vi "Create Object.vi"(11 "Ex Event Actor in":refnum<class "Ex Event Actor.lvclass">) -> (3 "Ex Event Actor out":refnum<class "Ex Event Actor.lvclass">)   [LabVIEW 2021, in "Ex Event Actor.lvclass"]
uses:
  Ex Event Actor.lvclass
  Ex Event Actor.lvclass/Ex Event Actor.ctl
  jettl/jettl.lvlib
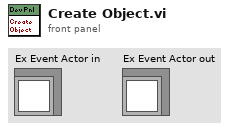
[diagram p1: front panel]
types:
  T1 = cluster{"Events":cluster{"Teardown":refnum<user-event>, "Pop Up":refnum<user-event>, "String Indicator":refnum<user-event>, "Button":refnum<user-event>}, "Refs":cluster{"FP Ref":refnum<vi>, "Pop Up":refnum<vi>, "String Indicator":refnum<vi>, "Button":refnum<vi>}, "BG Color":u32, "Event Actor":refnum<class "Event Actor.lvclass">}
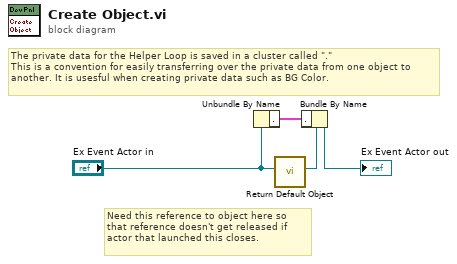
[diagram p0: block diagram]
diagram:
  # "The private data for the Helper Loop is saved in a cluster called \".\"\nThis is a convention for easily transferring over the private data from one object to another. It is usesful when creating private data such as BG Color."
  # "Need this reference to object here so that reference doesn't get released if actor that launched this closes."
  n1 = Unbundle By Name("Ex Event Actor in") -> ("."=w4:T1)
  n2 = call "Return Default Object.vi"("Object"="Ex Event Actor in") -> ("Default Object Instance"=w2:refnum<class "Ex Event Actor.lvclass">)  [unwired: 10 in]
  n3 = Bundle By Name(cluster=w2, "."=w4) -> (→"Ex Event Actor out":refnum<class "Ex Event Actor.lvclass">)
